vi "Set Temperature [°C].vi"(8 "error in (no error)":errorcluster, 10 "Temperature [°C]":dbl, 11 "CalibReport in":refnum<class "CalibReport.lvclass">) -> (0 "error out":errorcluster, 3 "CalibReport out":refnum<class "CalibReport.lvclass">)   [LabVIEW 2024, in "CalibReport.lvclass"]
uses:
  CalibReport.lvclass
  CalibReport.lvclass/CalibReport.ctl
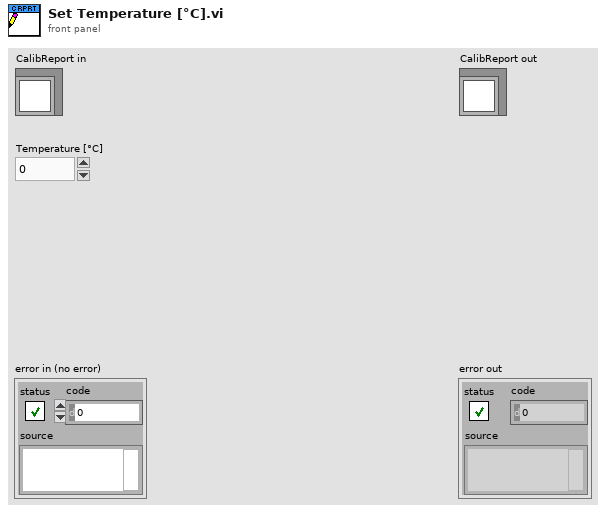
[diagram p1: front panel]
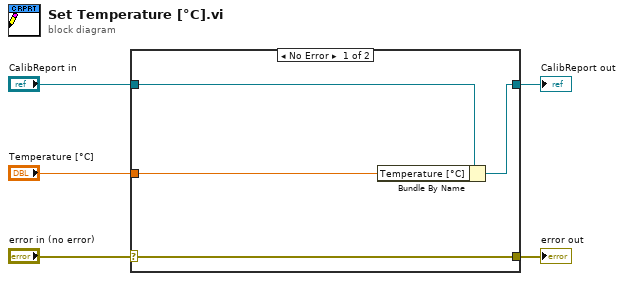
[diagram p0: block diagram]
diagram:
  n1 = case shown="No Error" "error in (no error)" {
    selector: "error in (no error)" -> [w9 w10]
    tunnel: [w9 w10] -> w4
    tunnel: [w7 w11] -> w2
    tunnel: "CalibReport in" -> [w8 w11]
    tunnel: "Temperature [°C]" -> [w6 _]
    frame No Error {
      n2 = Bundle By Name(cluster=w8, "Temperature [°C]"=w6) -> (w7:refnum<class "CalibReport.lvclass">)
    }
    frame Error {
    }
  }
  "error out" <- w4
  "CalibReport out" <- w2
